vi "FindTargetInSystemDefinition.vi"(8 "error in":errorcluster, 10 "target index":i32, 11 "system definition path":path) -> (0 "error out":errorcluster, 1 "Target":refnum<k39>, 2 "Root":refnum<k39>, 3 "System Definition":refnum<k39>)   [LabVIEW 2027, in "VeriStandTestUtilities.lvlib"]
uses:
  VeriStandTestUtilities.lvlib
  C:/NetCoreDLL/NationalInstruments.VeriStand.SystemDefinitionAPI.dll
  NetCoreDLL/NationalInstruments.VeriStand.SystemDefinitionAPI.dll
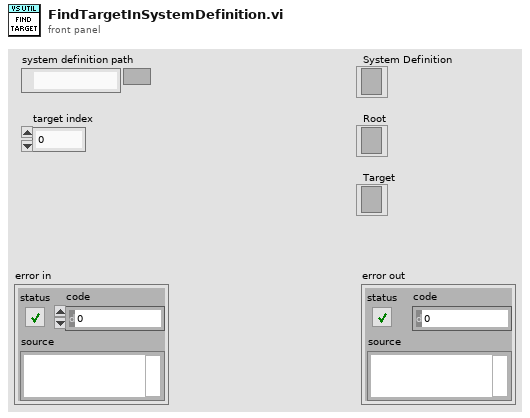
[diagram p1: front panel]
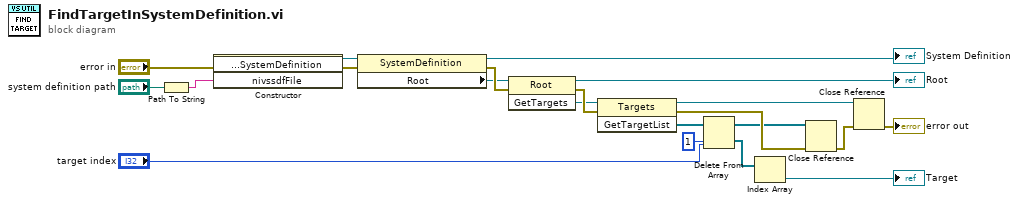
[diagram p0: block diagram]
diagram:
  n1 = Path To String(path="system definition path") -> (string=w20:string)
  n2 = constructor class="SystemDefinition"(error in="error in", "nivssdfFile"=w20) -> (reference out=w19:refnum<k39>, error out=w21:errorcluster)  [unwired: 2 in, 2 out]
  n3 = property class="SystemDefinition"(reference=w19, error in=w21) -> (reference out=→"System Definition":refnum<k39>, error out=w18:errorcluster, "Root"=w17:refnum<k39>)
  n4 = invoke class="Root" method="GetTargets"(reference=w17, error in=w18) -> (reference out=→"Root":refnum<k39>, error out=w16:errorcluster, "GetTargets"=w15:refnum<k39>)  [unwired: 1 in]
  n5 = invoke class="Targets" method="GetTargetList"(reference=w15, error in=w16) -> (reference out=w8:refnum<k39>, error out=w11:errorcluster, "GetTargetList"=w14:refnum<k39>[])  [unwired: 1 in]
  n6 = Delete From Array(array=w14, length=1, index="target index") -> (deleted portion=w7:refnum<k39>[], array with subset deleted=w10:refnum<k39>[])
  n7 = Index Array(array=w7) -> (element=→"Target":refnum<k39>)  [unwired: 1 in]
  n8 = Close Reference(reference=w10, error in (no error)=w11) -> (error out=w9:errorcluster)
  n9 = Close Reference(reference=w8, error in (no error)=w9) -> (error out=→"error out":errorcluster)
